vi "Deserialise content.vi"(8 "error in (no error)":errorcluster, 10 "JSON String to decode":string, 11 "object in":refnum<class "error Message.lvclass">) -> (0 "error out":errorcluster, 3 "object out":refnum<class "error Message.lvclass">)   [LabVIEW 2018, in "ClientMessaging.lvlib" / "error Message.lvclass"]
doc: "Convert content dictionary to class private data"
uses:
  error Message.lvclass
  c0b55c95-1b80-4604-8296-0b4dd3ac4bc8.vi
  2fe802b8-2bf6-4890-bfb7-9db01cbdcac4.vi
  88f9a830-f70e-47d6-ba70-474d34a1a121.vi
  Base Classes/Message Class/Message Class.lvclass
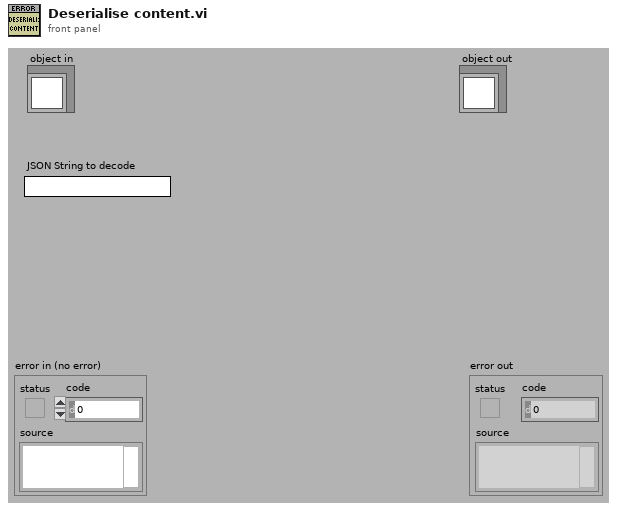
[diagram p1: front panel]
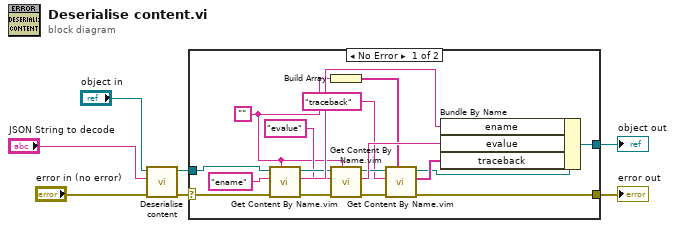
[diagram p0: block diagram]
diagram:
  n1 = call-parent "Deserialise content.vi"("error in (no error)"="error in (no error)", "JSON String to decode"="JSON String to decode", "object in"="object in") -> ("error out"=w1:errorcluster, "object out"=w4:refnum<class "error Message.lvclass">)  [unwired: 7 in]
  n2 = case shown="No Error" w1 {
    selector: w1 -> [w11 w26]
    tunnel: [w10 w26] -> w7
    tunnel: [w8 w25] -> w5
    tunnel: w4 -> [w24 w25]
    frame No Error {
      w18 = ""
      n3 = call "Get Content By Name.vim"("Type of content"=w18, "error in (no error)"=w11, "Name of Content Item"="ename" ("Element Name"), "Message In"=w24) -> ("error out"=w20:errorcluster, "Data Out"=w22:string, "Message Out"=w21:refnum<class "error Message.lvclass">)  [unwired: 5 in]
      n4 = Build Array(w18) -> (w13:string[])
      n5 = call "Get Content By Name.vim"("Type of content"=w18, "error in (no error)"=w20, "Name of Content Item"="evalue" ("Element Name"), "Message In"=w21) -> ("error out"=w15:errorcluster, "Data Out"=w17:string, "Message Out"=w16:refnum<class "error Message.lvclass">)  [unwired: 5 in]
      n6 = call "Get Content By Name.vim"("Type of content"=w13, "error in (no error)"=w15, "Name of Content Item"="traceback" ("Element Name"), "Message In"=w16) -> ("error out"=w10:errorcluster, "Data Out"=w12:string[], "Message Out"=w9:refnum<class "error Message.lvclass">)  [unwired: 5 in]
      n7 = Bundle By Name(cluster=w9, "ename"=w22, "evalue"=w17, "traceback"=w12) -> (w8:refnum<class "error Message.lvclass">)
    }
    frame Error {
    }
  }
  "error out" <- w7
  "object out" <- w5
